vi "Open Stimulator_individual_params.vi"(4 "error in (no error)":errorcluster, 5 "Stimulator Name":refnum<visa-resource-name>, 6 "timeout (ms)":u32=10000, 7 "Stimulator Mode":T2) -> (0 "error IO":errorcluster, 1 "Open Stim Result":T6, 2 "Stim Open":bool caption="Stim Open?", 3 "Stimulator":T1={"Log File In"=refnum, "Stimulator In"="", "Stimulator Mode"="", "Log Data"=FALSE, "Doublet/Triplet  Interval"=0.0, "Stim Frequency"=0.0, "N-Factor"=0, "Active Channels"=[], "Low-Frequency Channels"=[], "Stimulator State"=enum."Closed", "Mode Array"=[], "Current Array"=[], "Pulse Duration Array"=[], "VISA Timeout"=50})   [LabVIEW 2019]
uses:
  Controls/Stimulator Mode.ctl
  Controls/Stimulator Cluster.ctl
  Version 2/Data Type Defs/Pulse Mode (array).ctl
  Controls/Stim Current Array.ctl
  Controls/Pulse Duration Array.ctl
  Version 2/Data Type Defs/Obsolete/Stimulator Init Control_obs.ctl
  Version 2/Data Type Defs/Stim Init Data.ctl
  <vilib>/Instr/_visa.llb/VISA Configure Serial Port (Instr).vi
panel:
  out "VISA Configure Error (?)":errorcluster
  out "Open VISA Sesssions":refnum<visa-resource-name>[](array[refnum])
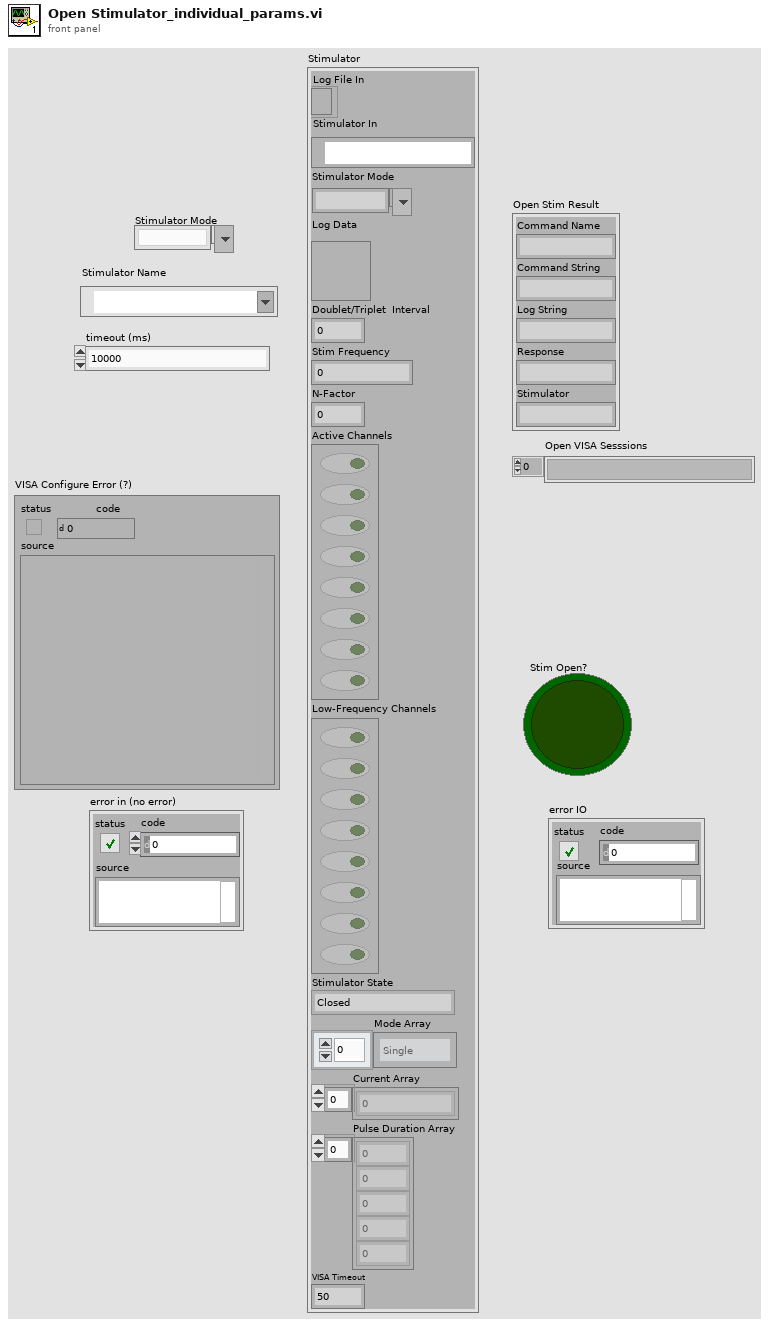
[diagram p1: front panel]
types:
  T1 = typedef "Stimulator Cluster.ctl" = cluster{"Log File In":refnum<file>, "Stimulator In":refnum<visa-resource-name>, "Stimulator Mode":T2, "Log Data":bool, "Doublet/Triplet  Interval":dbl, "Stim Frequency":dbl, "N-Factor":u8, "Active Channels":bool[], "Low-Frequency Channels":bool[], "Stimulator State":enum16{"Closed", "Open", "Initialized", "Stimulating"}, "Mode Array":T3, "Current Array":T4, "Pulse Duration Array":T5, "VISA Timeout":u32}
  T2 = typedef "Stimulator Mode.ctl" = string
  T3 = typedef "Pulse Mode (array).ctl" = enum16{"Single", "Doublet", "Triplet"}[]
  T4 = typedef "Stim Current Array.ctl" = u8[]
  T5 = typedef "Pulse Duration Array.ctl" = u32[]
  T6 = cluster{"Command Name":string, "Command String":string, "Log String":string, "Response":string, "Stimulator":string}
  T7 = typedef "Stimulator Init Control_obs.ctl" = cluster{"Stimulator Control":cluster{"Name":refnum<visa-resource-name>, "Mode":enum16{"LIVE", "SIM"}, "Visa Timeout":u32}, "Initialization Parameters":T8}
  T8 = typedef "Stim Init Data.ctl" = cluster{"Frequency":dbl, "N Factor":u8, "D/T Int":dbl, "Active Channels":bool[], "LF Channels":bool[]}
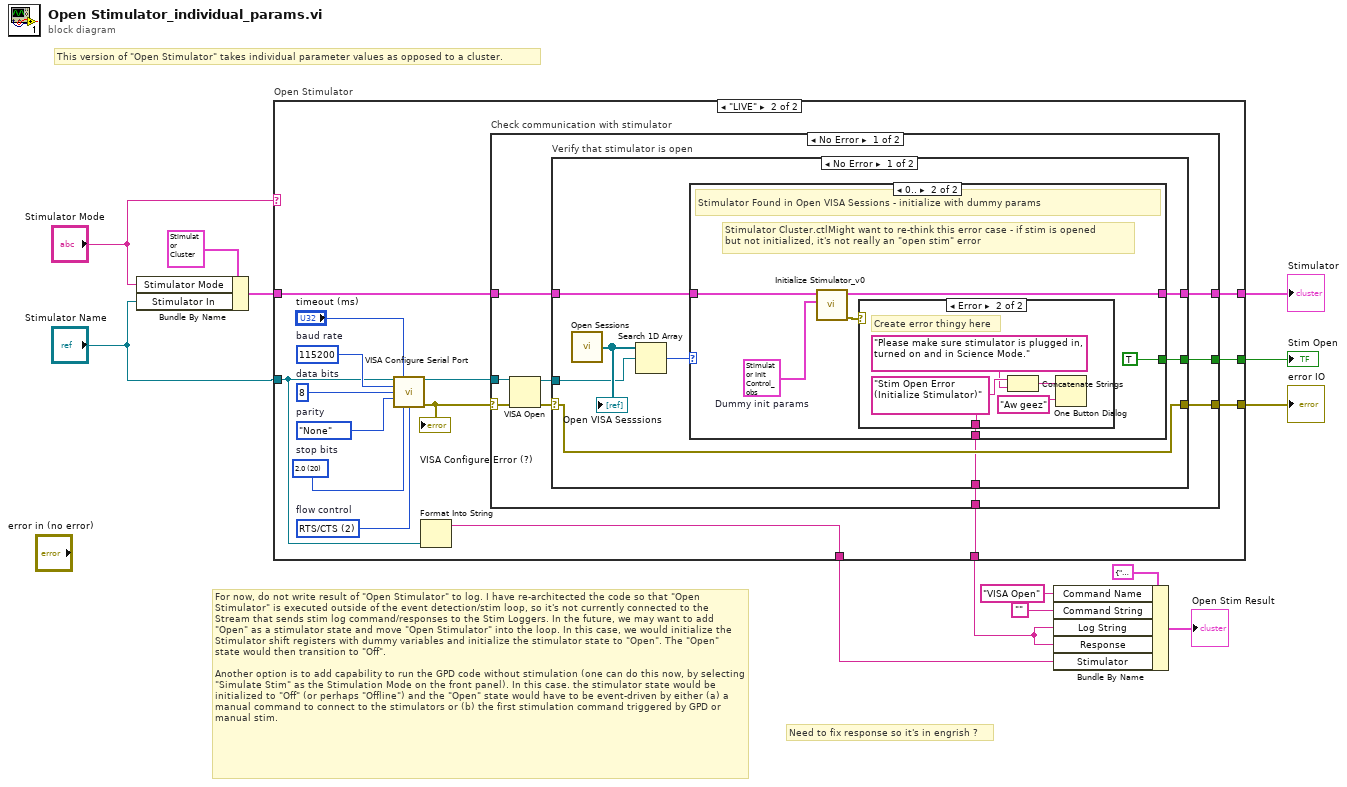
[diagram p0: block diagram]
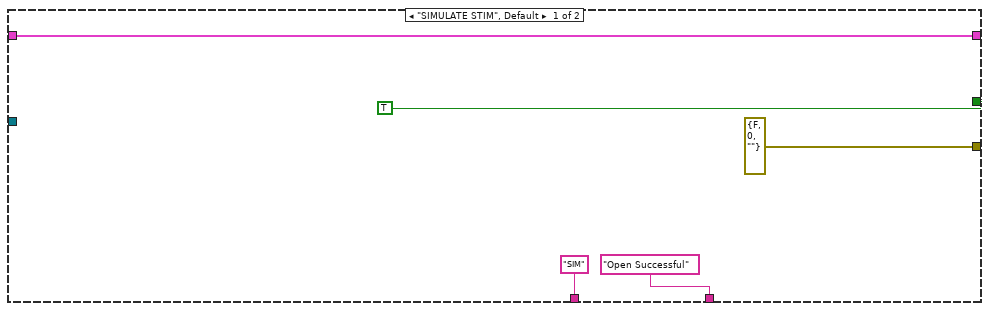
[diagram p2: hidden frame]
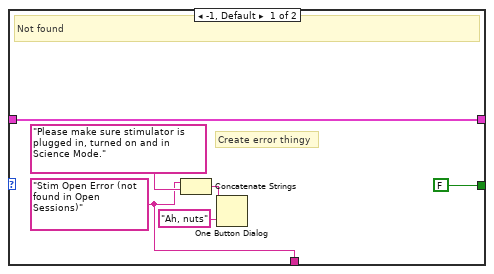
[diagram p3: hidden frame]
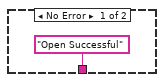
[diagram p4: hidden frame]
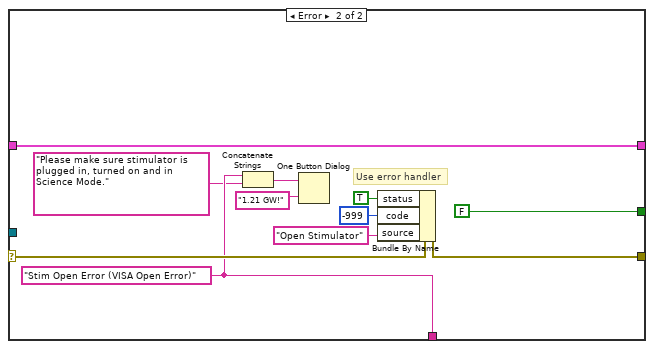
[diagram p5: hidden frame]
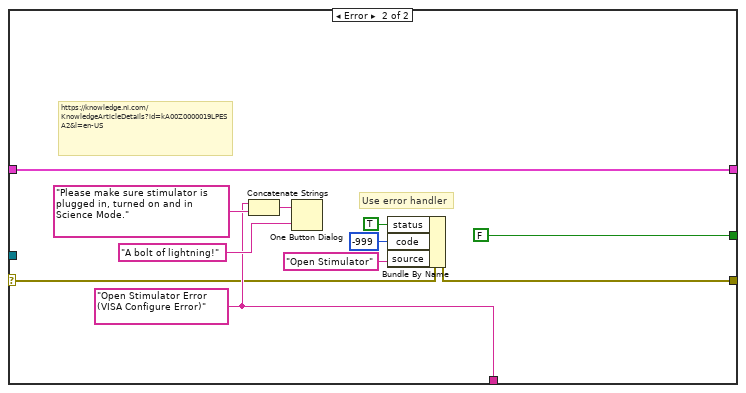
[diagram p6: hidden frame]
diagram:
  # "This version of \"Open Stimulator\" takes individual parameter values as opposed to a cluster."
  # "Need to fix response so it's in engrish ?"
  # "For now, do not write result of \"Open Stimulator\" to log. I have re-architected the code so that \"Open Stimulator\" is executed outside of the event detection/stim loop, so it's not currently connected to the Stream that sends stim log command/responses to the Stim Loggers. In the future, we may want to add \"Open\" as a stimulator state and move \"Open Stimulator\" into the loop. In this case, we would initialize the Stimulator shift registers with dummy variables and initialize the stimulator state to \"Open\". The \"Open\" state would then transition to \"Off\".\n\nAnother option is to add capability to run the GPD code without stimulation (one can do this now, by selecting \"Simulate Stim\" as the Stimulation Mode on the front panel). In this case. the stimulator state would be initialized to \"Off\" (or perhaps \"Offline\") and the \"Open\" state would have to be event-driven by either (a) a manual command to connect to the stimulators or (b) the first stimulation command triggered by GPD or manual stim."
  n1 = Bundle By Name(cluster=T1 {"Log File In"=refnum, "Stimulator In"="", "Stimulator Mode"="", "Log Data"=FALSE, "Doublet/Triplet  Interval"=0.0, "Stim Frequency"=0.0, "N-Factor"=0, "Active Channels"=[], "Low-Frequency Channels"=[], "Stimulator State"=enum."Closed", "Mode Array"=[], "Current Array"=[], "Pulse Duration Array"=[], "VISA Timeout"=0} ("New Stimulator"), "Stimulator Mode"="Stimulator Mode", "Stimulator In"="Stimulator Name") -> (w3:T1)
  n2 = case "Open Stimulator" shown="\"LIVE\"" "Stimulator Mode" {
    tunnel: [TRUE w25] -> w13
    tunnel: [errorcluster {"status"=FALSE, "code"=0, "source"=""} ("error IO") w24] -> w12
    tunnel: [w14 w23] -> w1
    tunnel: ["Open Successful" w22] -> w6
    tunnel: ["SIM" w21] -> w8
    tunnel: "Stimulator Name" -> [_ w20]
    tunnel: w3 -> [w14 w19]
    frame "SIMULATE STIM", Default {
    }
    frame "LIVE" {
      w29 = u16 2 items=["None", "XON/XOFF", "RTS/CTS", "XON/XOFF & RTS/CTS", "DTR/DSR", "XON/XOFF & DTR/DSR"]  # flow control
      w30 = u16 20 items=["1.0"=10, "1.5"=15, "2.0"=20]  # stop bits
      w31 = enum16{"None", "Odd", "Even", "Mark", "Space"}."None"  # parity
      w32 = u16 8  # data bits
      w33 = u32 115200  # baud rate
      n3 = call-poly "VISA Configure Serial Port"("VISA resource name"=w20, "timeout (10sec)"="timeout (ms)", "baud rate (9600)"=w33, "data bits (8)"=w32, "parity (0:none)"=w31, "stop bits (10: 1 bit)"=w30, "flow control (0:none)"=w29) -> ("VISA resource name out"=w26:refnum<visa-resource-name>, "error out"=w27:errorcluster)  [unwired: 7 in]
      "VISA Configure Error (?)" <- w27
      n4 = Format Into String(w20) -> (resulting string=w21:string)  [unwired: 3 in, 1 out]
      n5 = case "Check communication with stimulator" shown="No Error" w27 {
        selector: w27 -> [w38 w81]
        tunnel: w26 -> [w40 _]
        tunnel: [w39 FALSE] -> w25
        tunnel: [w37 w80] -> w24
        tunnel: [w36 w85] -> w22
        tunnel: [w35 w79] -> w23
        tunnel: w19 -> [w34 w79]
        frame No Error {
          n6 = VISA Open(error in (no error)=w38, VISA resource name=w40) -> (VISA resource name=w42:refnum<visa-resource-name>, error out=w41:errorcluster)  [unwired: 3 in]
          n7 = case "Verify that stimulator is open" shown="No Error" w41 {
            selector: w41 -> [w49 w74]
            tunnel: [w49 w73] -> w37
            tunnel: w42 -> [w44 _]
            tunnel: [w48 FALSE] -> w39
            tunnel: [w46 w71] -> w36
            tunnel: [w45 w68] -> w35
            tunnel: w34 -> [w43 w68]
            frame No Error {
              n8 = call <vilib>:"Open Sessions.vi"() -> ("Array of Refnums"=w47:refnum<visa-resource-name>[])  [unwired: 2 in]
              "Open VISA Sesssions" <- w47
              n9 = Search 1D Array(1D array=w47, element=w44) -> (index of element=w50:i32)  [unwired: 1 in]
              n10 = case shown="0.." w50 {
                tunnel: [FALSE ("Stim Open") TRUE ("Stim Open")] -> w48
                tunnel: [w52 w61] -> w46
                tunnel: [w51 w59] -> w45
                tunnel: w43 -> [w51 w57]
                frame -1, Default {
                  w52 = "Stim Open Error (not found in Open Sessions)"
                  # "Create error thingy"
                  # "Not found"
                  n11 = Concatenate Strings(w52, "Please make sure stimulator is plugged in, turned on and in Science Mode." ("message")) -> (w53:string)
                  n12 = One Button Dialog(message=w53, button name ("OK")="Ah, nuts") -> ()  [unwired: 1 out]
                }
                frame 0.. {
                  w60 = T7 {"Stimulator Control"={"Name"="", "Mode"=enum."SIM", "Visa Timeout"=0}, "Initialization Parameters"={"Frequency"=0.0, "N Factor"=0, "D/T Int"=0.0, "Active Channels"=[TRUE, TRUE, TRUE, TRUE, TRUE], "LF Channels"=[FALSE, FALSE, FALSE, FALSE, FALSE]}}  # Dummy init params
                  # "Stimulator Cluster.ctlMight want to re-think this error case - if stim is opened \nbut not initialized, it's not really an \"open stim\" error"
                  # "Stimulator Found in Open VISA Sessions - initialize with dummy params"
                  n13 = call "Initialize Stimulator_v0.vi"("Initialization Parameters"=w60, "Stimulator"=w57) -> ("error out"=w58:errorcluster, "Stimulator Out"=w59:T1)  [unwired: 2 in, 2 out]
                  n14 = case shown="Error" w58 {
                    tunnel: ["Open Successful" w66] -> w61
                    frame No Error {
                    }
                    frame Error {
                      w66 = "Stim Open Error (Initialize Stimulator)"
                      # "Create error thingy here"
                      n15 = Concatenate Strings(w66, "Please make sure stimulator is plugged in, turned on and in Science Mode." ("message")) -> (w64:string)
                      n16 = One Button Dialog(message=w64, button name ("OK")="Aw geez") -> ()  [unwired: 1 out]
                    }
                  }
                }
              }
            }
            frame Error {
              w71 = "Stim Open Error (VISA Open Error)"
              # "Use error handler"
              n17 = Concatenate Strings(w71, "Please make sure stimulator is plugged in, turned on and in Science Mode." ("message")) -> (w69:string)
              n18 = One Button Dialog(message=w69, button name ("OK")="1.21 GW!") -> ()  [unwired: 1 out]
              n19 = Bundle By Name(cluster=w74, "status"=TRUE, "code"=-999, "source"="Open Stimulator") -> (w73:errorcluster)
            }
          }
        }
        frame Error {
          w85 = "Open Stimulator Error (VISA Configure Error)"
          # "Use error handler"
          # "https://knowledge.ni.com/KnowledgeArticleDetails?id=kA00Z0000019LPESA2&l=en-US"
          n20 = Concatenate Strings(w85, "Please make sure stimulator is plugged in, turned on and in Science Mode." ("message")) -> (w87:string)
          n21 = One Button Dialog(message=w87, button name ("OK")="A bolt of lightning!") -> ()  [unwired: 1 out]
          n22 = Bundle By Name(cluster=w81, "status"=TRUE, "code"=-999, "source"="Open Stimulator") -> (w80:errorcluster)
        }
      }
    }
  }
  "error IO" <- w12
  "Stim Open" <- w13
  "Stimulator" <- w1
  n23 = Bundle By Name(cluster=T6 {"Command Name"="Command Name", "Command String"="Command String", "Log String"="Log String", "Response"="Response", "Stimulator"="Stimulator"} ("Cluster"), "Command Name"="VISA Open", "Command String"="", "Log String"=w6, "Response"=w6, "Stimulator"=w8) -> (→"Open Stim Result":T6)
